vi "UI.progressbar.vi"(7 "write?":bool, 8 "error in":errorcluster, 9 "Value":u8, 10 "Maximum":dbl, 11 "Slide in":refnum<vi>) -> (0 "error out":errorcluster)   [LabVIEW 2020]
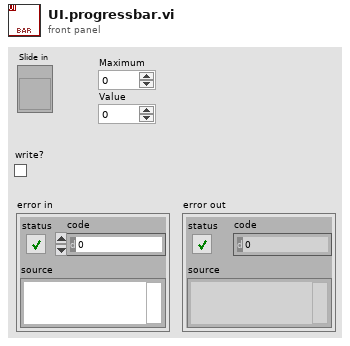
[diagram p1: front panel]
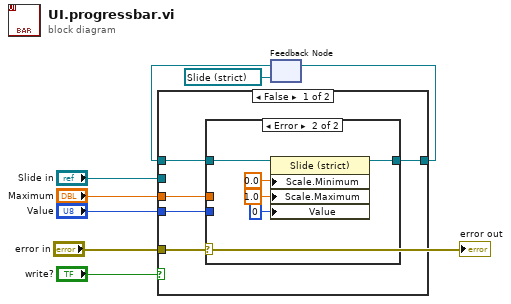
[diagram p0: block diagram]
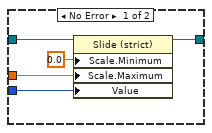
[diagram p2: hidden frame]
diagram:
  n1 = feedback #1(refnum<vi> refnum ("Slide in")) -> (w5:refnum<vi>)
  n2 = case shown="False" "write?" {
    tunnel: "Slide in" -> [_ w24]
    tunnel: w5 -> [w13 _]
    tunnel: [w12 w24] -> w6
    tunnel: "Value" -> [w11 _]
    tunnel: "Maximum" -> [w10 _]
    tunnel: "error in" -> [w9 _]
    frame False {
      n3 = case shown="Error" w9 {
        tunnel: w13 -> [w18 w23]
        tunnel: [w17 w22] -> w12
        tunnel: w11 -> [w15 _]
        tunnel: w10 -> [w14 _]
        frame No Error {
          n4 = property class="Slide (strict)"(reference=w18, "Scale.Minimum"=0.0 ("Scale.Range:Minimum"), "Scale.Maximum"=w14, "Value"=w15) -> (reference out=w17:refnum<vi>)  [unwired: 1 in, 1 out]
        }
        frame Error {
          n5 = property class="Slide (strict)"(reference=w23, "Scale.Minimum"=0.0 ("Scale.Range:Minimum"), "Scale.Maximum"=1.0 ("Scale.Range:Maximum"), "Value"=u8 0) -> (reference out=w22:refnum<vi>)  [unwired: 1 in, 1 out]
        }
      }
    }
    frame True {
    }
  }
  n6 = feedback-in #1(w6) -> ()
  "error out" <- "error in"
